vi "GetRFc1Cal.vi"(6 "Legacy (f)?":bool, 7 "Step Size (0 = default)":dbl, 8 "error in (no error)":errorcluster, 10 "Freq Range":dbl[](array[numeric])) -> (0 "error out":errorcluster, 2 "C1 Cal Data":dbl[](array[numeric]))   [LabVIEW 2011]
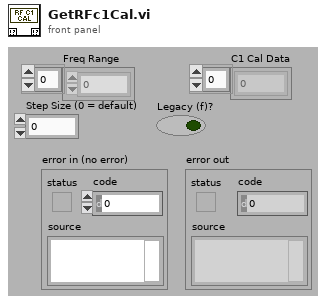
[diagram p1: front panel]
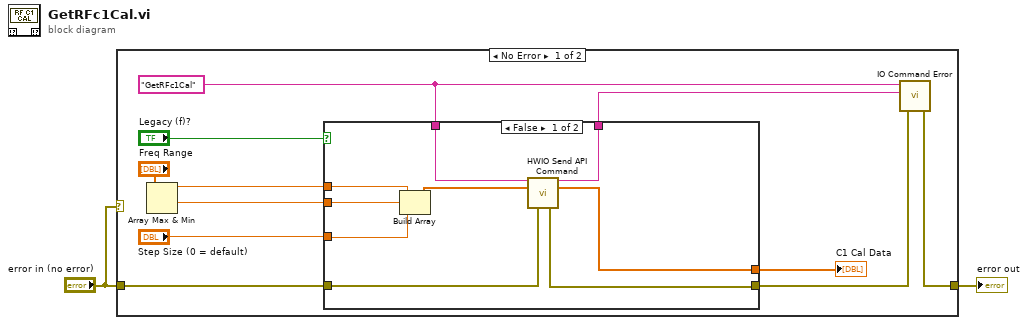
[diagram p0: block diagram]
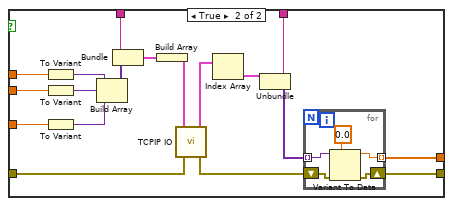
[diagram p2: hidden frame]
diagram:
  n1 = case shown="No Error" "error in (no error)" {
    tunnel: "error in (no error)" -> [w13 w46]
    tunnel: [w11 w46] -> w2
    frame No Error {
      w9 = "GetRFc1Cal"
      n2 = Array Max & Min(array="Freq Range") -> (max value=w6:dbl, min value=w5:dbl)  [unwired: 2 out]
      n3 = case shown="False" "Legacy (f)?" {
        tunnel: w13 -> [w19 w39]
        tunnel: [w20 w38] -> w12
        tunnel: [w21 w37] -> w10
        tunnel: w9 -> [w22 w36]
        tunnel: [w18 w29] -> w7
        tunnel: w6 -> [w17 w28]
        tunnel: w5 -> [w16 w27]
        tunnel: "Step Size (0 = default)" -> [w15 w26]
        frame False {
          n4 = Build Array(w17, w16, w15) -> (w14:dbl[])
          n5 = call "HWIO Send API Command.vi"("Action"=w22, "Double"=w14, "error in (no error)"=w19) -> ("Action out"=w21:string, "Double out"=w18:dbl[], "error out"=w20:errorcluster)  [unwired: 5 in, 5 out]
        }
        frame True {
          n6 = To Variant(anything=w28) -> (Variant=w24:variant)
          n7 = To Variant(anything=w27) -> (Variant=w31:variant)
          n8 = To Variant(anything=w26) -> (Variant=w25:variant)
          n9 = Build Array(w24, w31, w25) -> (w32:variant[])
          n10 = Bundle(w36, w32) -> (w40:cluster{string, variant[]})  [unwired: 1 out]
          n11 = Build Array(w40) -> (w33:cluster{string, variant[]}[])
          n12 = call "TCPIP IO.vi"("error in (no error)"=w39, "Commands"=w33) -> ("error out"=w23:errorcluster, "Responses"=w35:cluster{string, variant[]}[])  [unwired: 1 in, 3 out]
          n13 = Index Array(array=w35) -> (element=w34:cluster{string, variant[]})  [unwired: 1 in]
          n14 = Unbundle(w34) -> (w37:string, w30:variant[])
          n15 = for {
            shift-right: [w44] -> w38
            shift-left: w23 -> [w45]
            tunnel: w30 -> [w42] mode=indexing
            tunnel: [w41] -> w29 mode=indexing
            n16 = Variant To Data(error in=w45, type=0.0 ("Injected Power, dBm"), Variant=w42) -> (data=w41:dbl, error out=w44:errorcluster)
          }
        }
      }
      "C1 Cal Data" <- w7
      n17 = call "IO Command Error.vi"("error in (no error)"=w12, "Command Returned (\"\")"=w10, "Command Sent (\"\")"=w9) -> ("error out"=w11:errorcluster)  [unwired: 4 out]
    }
    frame Error {
    }
  }
  "error out" <- w2
